vi "display.vi"(8 "error in (no error)":errorcluster, 11 "GeneralDisplay in":refnum<class "GeneralDisplay.lvclass">) -> (0 "error out":errorcluster, 3 "GeneralDisplay out":refnum<class "GeneralDisplay.lvclass">)   [LabVIEW 2017, in "GeneralDisplay.lvclass"]
uses:
  GeneralDisplay.lvclass
panel:
  out "Pressure":dbl(knob) scale=0.0..10.0
  out "Humidity":dbl(slide) scale=0.0..10.0
  out "Temperature":dbl(slide) scale=0.0..10.0
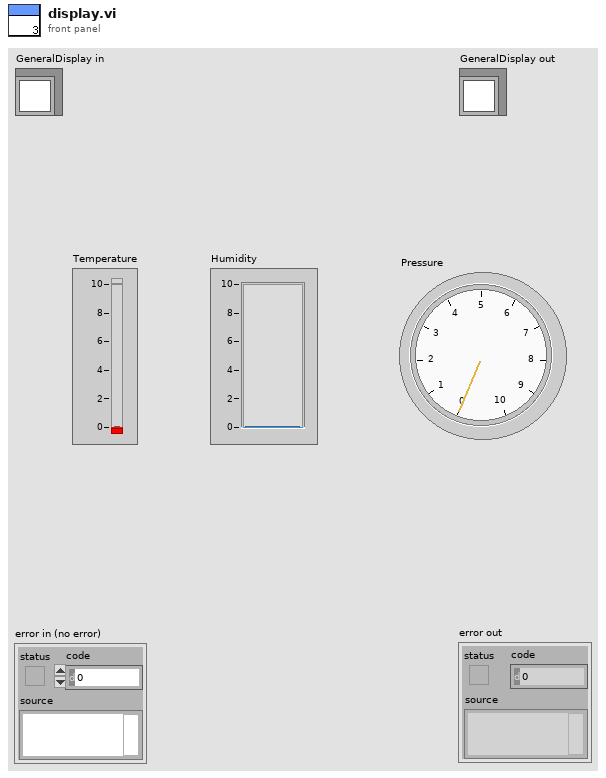
[diagram p1: front panel]
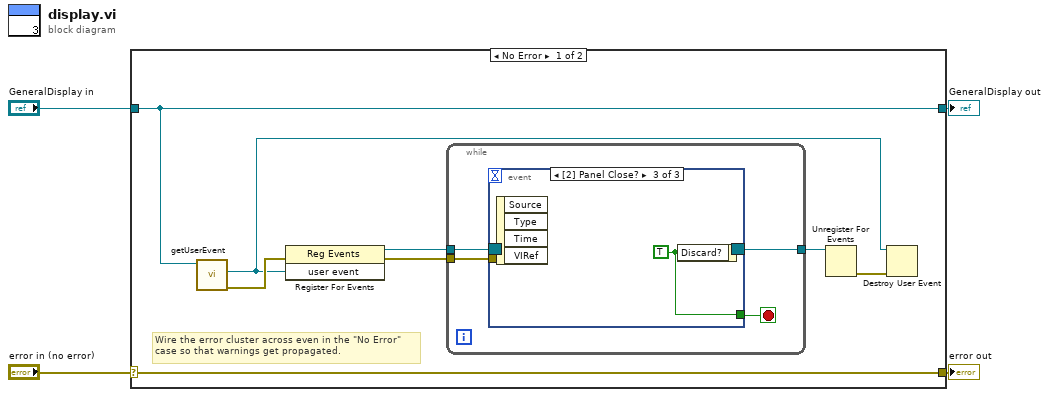
[diagram p0: block diagram]
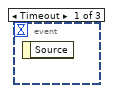
[diagram p2: hidden frame]
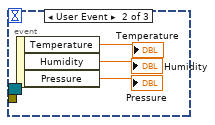
[diagram p3: hidden frame]
diagram:
  n1 = case shown="No Error" "error in (no error)" {
    selector: "error in (no error)" -> [w12 w22]
    tunnel: [w12 w22] -> w3
    tunnel: [w8 w21] -> w1
    tunnel: "GeneralDisplay in" -> [w8 w21]
    frame No Error {
      # "Wire the error cluster across even in the \"No Error\"\ncase so that warnings get propagated."
      n2 = call-dynamic "getUserEvent.vi"("GeneralDisplay in"=w8) -> ("error out"=w10:errorcluster, "user event"=w5:refnum<user-event>)  [unwired: 8 in, 1 out]
      n3 = register-events(error in=w10, w5) -> (reference out=w11:refnum<event-registration>, error out=w9:errorcluster)  [unwired: 1 in]
      n4 = while {
        tunnel: w11 -> [w16]
        tunnel: w9 -> [w15]
        tunnel: [w13] -> w7
        stop <- w14 stop-if-true
        n5 = event shown="[2] Panel Close?" {
          selector: w16 -> [_ _ _]
          dyn-events: [_ _ _] -> w13
          timeout: _ -> [_ _ _]
          tunnel: w15 -> [_ _ _]
          tunnel: [_ _ w20] -> w14
          event Timeout {
            n6 = event-data() -> ()  [unwired: 1 in, 1 out]
          }
          event User Event {
            n7 = event-data() -> ("Temperature"=→"Temperature":dbl, "Humidity"=→"Humidity":dbl, "Pressure"=→"Pressure":dbl)  [unwired: 1 in]
          }
          event Panel Close? {
            w20 = TRUE ("Discard?")
            n8 = event-data() -> ()  [unwired: 1 in, 4 out]
            n9 = event-data("Discard?"=w20) -> ()  [unwired: 1 in, 1 out]
          }
        }
      }
      n10 = Unregister For Events(event registration refnum=w7) -> (error out=w6:errorcluster)  [unwired: 1 in]
      n11 = Destroy User Event(user event=w5, error in=w6) -> ()  [unwired: 1 out]
    }
    frame Error {
    }
  }
  "error out" <- w3
  "GeneralDisplay out" <- w1
